vi "TCP Read with Length (TCP Cluster).vi"(8 "error in (no error)":errorcluster, 9 "Timeout":i32, 11 "connection ID":refnum<k5>) -> (0 "error out":errorcluster, 1 "Timeout?":bool, 2 "TCP Cluster":T1={"Datatype"=enum."Message", "String"="Send to sobot"}, 3 "connection ID out":refnum<k5>)   [LabVIEW 2017]
uses:
  TypeDefinitions/TCP Cluster.ctl
  TypeDefinitions/TCP Commands.ctl
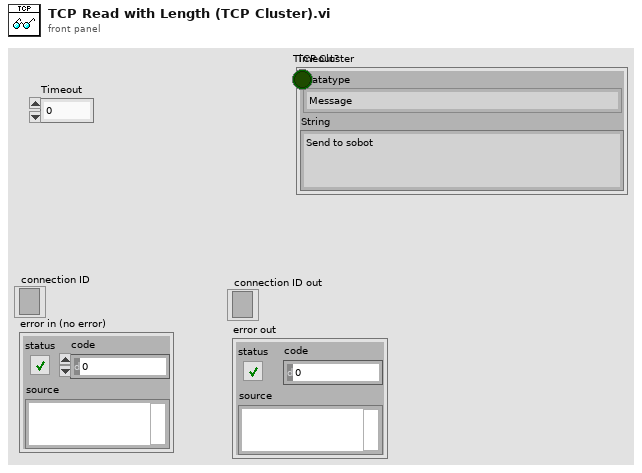
[diagram p1: front panel]
types:
  T1 = typedef "TCP Cluster.ctl" = cluster{"Datatype":T2, "String":string}
  T2 = typedef "TCP Commands.ctl" = enum16{"Timeout", "Log", "Message", "ManualDrive", "Stop", "Command"}
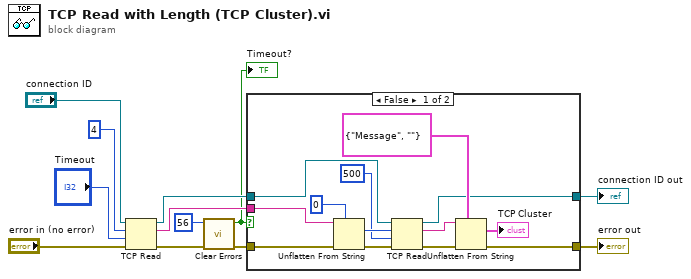
[diagram p0: block diagram]
diagram:
  n1 = TCP Read(connection ID="connection ID", bytes to read=4, error in (no error)="error in (no error)", 9:"Timeout") -> (connection ID out=w10:refnum<k5>, data out=w11:string, error out=w5:errorcluster)  [unwired: 1 in]
  n2 = call <vilib>:"Clear Errors.vi"("error in (no error)"=w5, "specific error code to clear (0: all)"=56) -> ("error out"=w4:errorcluster, "specific error cleared?"=w2:bool)  [unwired: 4 in]
  "Timeout?" <- w2
  n3 = case shown="False" w2 {
    tunnel: w11 -> [w25 _]
    tunnel: w10 -> [w19 w27]
    tunnel: [w15 w26] -> w6
    tunnel: w4 -> [w14 w26]
    tunnel: [w13 w27] -> w1
    frame False {
      n4 = Unflatten From String(type=0 ("bytes to read"), binary string=w25, error in (no error)=w14) -> (value=w23:i32, error out=w22:errorcluster)  [unwired: 2 in, 1 out]
      n5 = TCP Read(connection ID=w19, bytes to read=w23, error in (no error)=w22, 9:500 ("timeout ms (25000)")) -> (connection ID out=w13:refnum<k5>, data out=w21:string, error out=w20:errorcluster)  [unwired: 1 in]
      n6 = Unflatten From String(type=T1 {"Datatype"=enum."Message", "String"=""}, binary string=w21, error in (no error)=w20) -> (value=→"TCP Cluster":T1, error out=w15:errorcluster)  [unwired: 2 in, 1 out]
    }
    frame True {
    }
  }
  "error out" <- w6
  "connection ID out" <- w1
